vi "CheckCore.vi"(8 "error in (no error)":errorcluster, 9 "# of Refs":i32, 10 "References":refnum<vi>[](array[refnum]), 11 "Property in":refnum<class "Property.lvclass">) -> (0 "error out":errorcluster, 1 "Reject?":bool, 2 "dup References":refnum<vi>[](array[refnum]), 3 "Property out":refnum<class "Property.lvclass">)   [LabVIEW 2014, in "lvbuildsecurity.lvlib" / "Property.lvclass"]
uses:
  Property.lvclass
  Blacklist.lvclass/Blacklist.ctl
  ReadVIRefnum.vi
  ReadCLI.vi
  ReadItems.vi
  <vilib>/Wiresmith Technology/LabVIEW CLI/CLI Class/CLI.lvclass
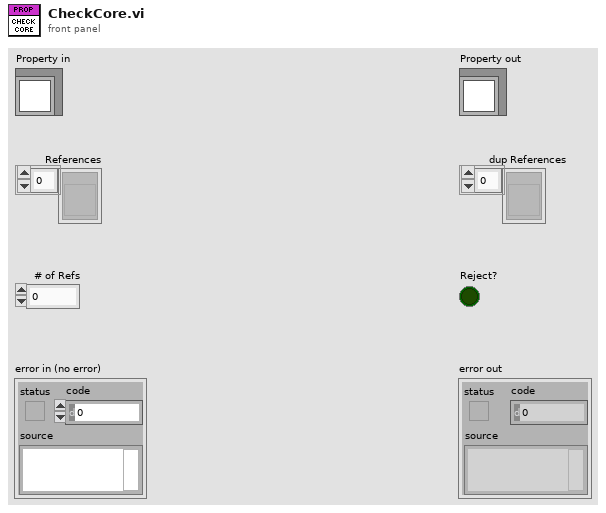
[diagram p1: front panel]
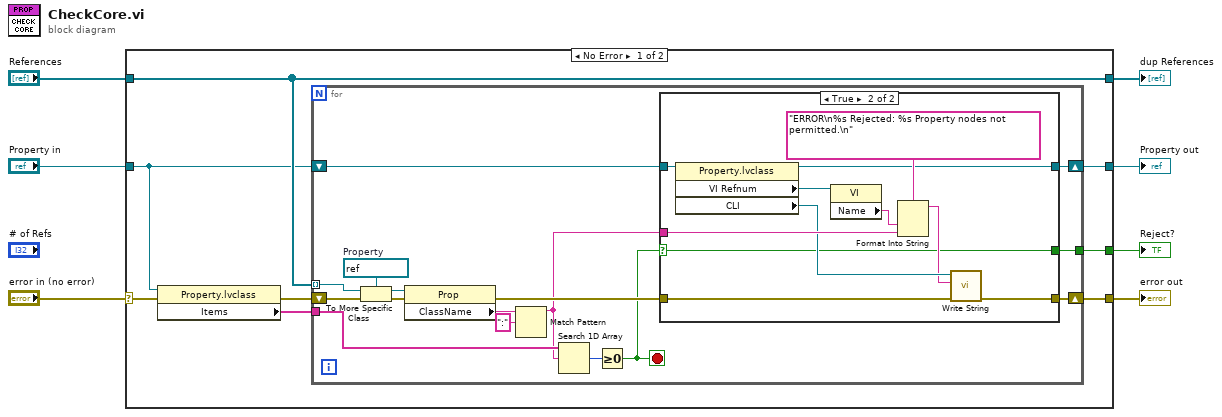
[diagram p0: block diagram]
diagram:
  n1 = case shown="No Error" "error in (no error)" {
    selector: "error in (no error)" -> [w13 w48]
    tunnel: [w15 w48] -> w2
    tunnel: "References" -> [w14 w46]
    tunnel: "Property in" -> [w9 w47]
    tunnel: [w8 w47] -> w6
    tunnel: [w14 w46] -> w5
    tunnel: [w10 _] -> w1
    frame No Error {
      n2 = property class="Property.lvclass"(reference=w9, error in=w13) -> (error out=w12:errorcluster, "Items"=w11:string[])  [unwired: 1 out]
      n3 = for {
        tunnel: w14 -> [w30] mode=indexing
        shift-right: [w21] -> w15
        shift-left: w12 -> [w31]
        tunnel: w11 -> [w26]
        tunnel: [w20] -> w10
        shift-right: [w16] -> w8
        shift-left: w9 -> [w17]
        stop <- w19 stop-if-true
        w29 = refnum<vi> refnum  # Property
        n4 = To More Specific Class(target class=w29, reference=w30, error in=w31) -> (specific class reference=w27:refnum<vi>, error out=w28:errorcluster)
        n5 = property class="Prop"(reference=w27, error in=w28) -> (error out=w22:errorcluster, "ClassName"=w24:string)  [unwired: 1 out]
        n6 = Match Pattern(string=w24, regular expression=":") -> (before substring=w18:string)  [unwired: 1 in, 3 out]
        n7 = Search 1D Array(1D array=w26, element=w18) -> (index of element=w25:i32)  [unwired: 1 in]
        n8 = Greater Or Equal To 0?(x=w25) -> (x >= 0?=w19:bool)
        n9 = case shown="True" w19 {
          selector: w19 -> [w32 w35]
          tunnel: w17 -> [w34 w45]
          tunnel: [w34 w38] -> w16
          tunnel: w18 -> [_ w41]
          tunnel: w22 -> [w33 w37]
          tunnel: [w33 w36] -> w21
          tunnel: [w32 w35] -> w20
          frame False {
          }
          frame True {
            n10 = property class="Property.lvclass"(reference=w45) -> (reference out=w38:refnum<class "Property.lvclass">, "VI Refnum"=w43:refnum<vi>, "CLI"=w40:refnum<class "CLI.lvclass">)  [unwired: 1 in, 1 out]
            n11 = property class="VI"(reference=w43) -> ("Name"=w42:string)  [unwired: 1 in, 2 out]
            n12 = Format Into String(format string="ERROR\n%s Rejected: %s Property nodes not permitted.\n", w42, w41) -> (resulting string=w39:string)  [unwired: 2 in, 1 out]
            n13 = call <vilib>:"Write String.vi"("error in (no error)"=w37, "Text to Write"=w39, "CLI in"=w40) -> ("error out"=w36:errorcluster)  [unwired: 7 in, 1 out]
          }
        }
      }
    }
    frame Error {
    }
  }
  "error out" <- w2
  "Property out" <- w6
  "dup References" <- w5
  "Reject?" <- w1
